vi "CAD@DelPart__Parameter.vi"(1 "ParamterIn":string) -> (0 "ParamterOut":string)   [LabVIEW 2020]
panel:
  out "Part Name":string[](array[string])
  in  "PartName":string(combo)
  in  "Confirm":bool
  # "CAD@DelPart $Part1(,$Part2,$Part3,......)"
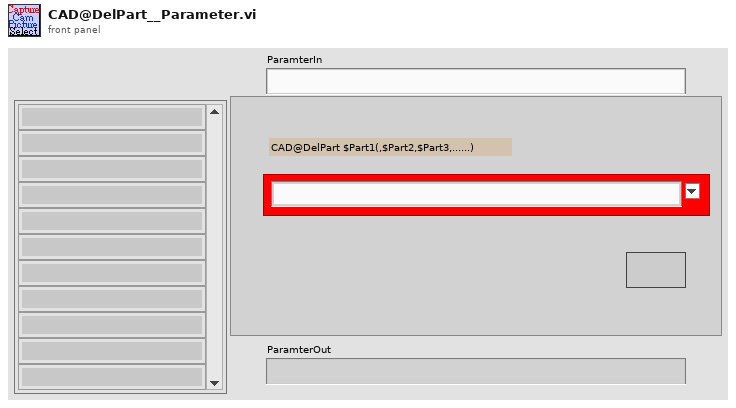
[diagram p1: front panel]
types:
  T1 = enum16{"Init", "Load Tool", "Load Part", "Get Tool Property", "Get Part Property", "Set Tool to End Matrix", "Set Part to Tool Matrix", "Calculate Part to Tool & End Matrix", "Create Part From Copy", "Delete Part", "Create Part From Step File"}
  T2 = cluster{"Tool Name":string[], "Part Name":string[]}
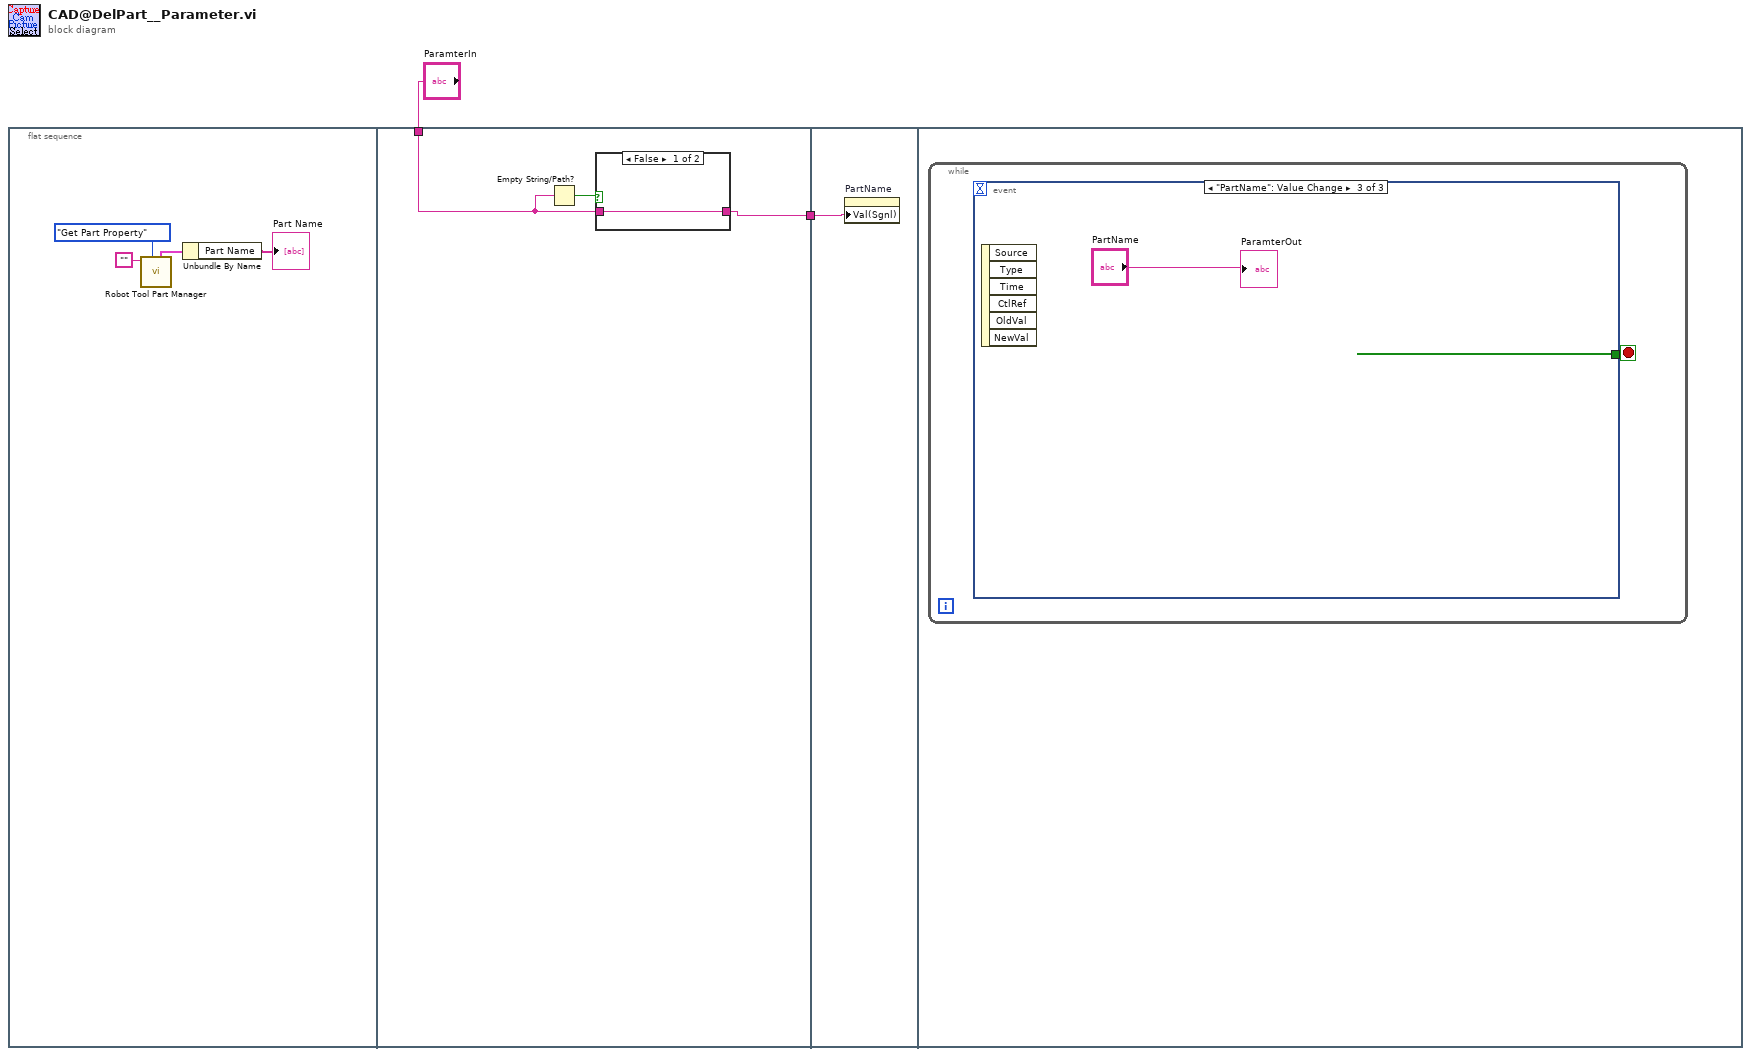
[diagram p0: block diagram]
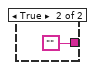
[diagram p2: hidden frame]
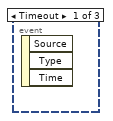
[diagram p3: hidden frame]
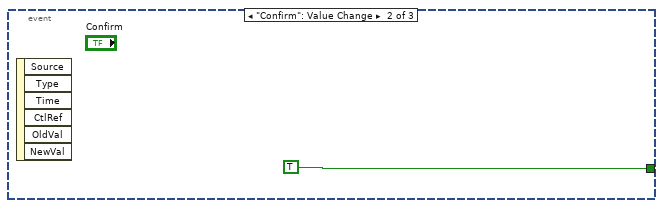
[diagram p4: hidden frame]
diagram:
  n1 = flat-sequence {
    tunnel: "ParamterIn" -> [w7]
    tunnel: [w8] -> w1
    tunnel: w1 -> [w12]
    frame #0 {
      n2 = call "Robot Tool Part Manager.vi"("CMD"=T1."Get Part Property", "Tool / Part Name"="") -> ("NameList"=w4:T2)  [unwired: 4 in, 5 out]
      n3 = Unbundle By Name(w4) -> ("Part Name"=→"Part Name":string[])
    }
    frame #1 {
      n4 = Empty String/Path?(string/path=w7) -> (empty?=w9:bool)
      n5 = case shown="False" w9 {
        tunnel: w7 -> [w10 _]
        tunnel: [w10 ""] -> w8
        frame False {
        }
        frame True {
        }
      }
    }
    frame #2 {
      n6 = property on="PartName" class="CmbBox"("Val(Sgnl)"=w12) -> ()  [unwired: 2 in, 2 out]
    }
    frame #3 {
      n7 = while {
        stop <- w13 stop-if-true
        n8 = event shown="[2] \"PartName\": Value Change" {
          selector: _ -> [_ _ _]
          dyn-events: _ -> [_ _ _]
          timeout: _ -> [_ _ _]
          tunnel: [_ TRUE _] -> w13
          event Timeout {
            n9 = event-data() -> ()  [unwired: 1 in, 3 out]
          }
          event "Confirm": Value Change {
            n10 = event-data() -> ()  [unwired: 1 in, 6 out]
          }
          event "PartName": Value Change {
            n11 = event-data() -> ()  [unwired: 1 in, 6 out]
            "ParamterOut" <- "PartName"
          }
        }
      }
    }
  }
